vi "Get Trigger Source.vi"(8 "error in":errorcluster, 11 "VISA resource name in":refnum<visa-resource-name>) -> (0 "error out":errorcluster, 2 "Trigger Source":string, 3 "VISA resource name out":refnum<visa-resource-name>)   [LabVIEW 2021, in "Keysight U1282A.lvlib"]
doc: "El comando obtener fuente de disparo (TRIG:SOUR?) regresa el tipo de fuente de disparo."
uses:
  Keysight U1282A.lvlib
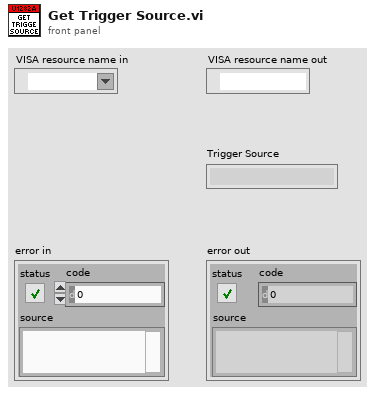
[diagram p1: front panel]
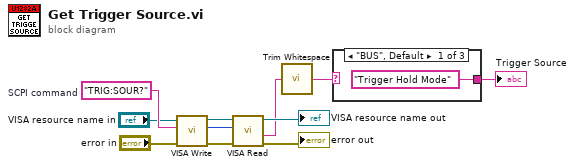
[diagram p0: block diagram]
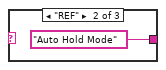
[diagram p2: hidden frame]
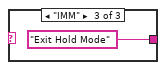
[diagram p3: hidden frame]
diagram:
  w4 = "TRIG:SOUR?"  # SCPI command
  n1 = call "VISA Write.vi"("error in"="error in", "SCPI command"=w4, "VISA resource in"="VISA resource name in") -> ("error out"=w11:errorcluster, "Bytes at Port out"=w9:u32, "VISA resource out"=w10:refnum<visa-resource-name>)  [unwired: 6 in]
  n2 = call "VISA Read.vi"("error in"=w11, "Bytes at Port in"=w9, "VISA resource in"=w10) -> ("error out"=→"error out":errorcluster, "Reading"=w3:string, "VISA resource out"=→"VISA resource name out":refnum<visa-resource-name>)  [unwired: 5 in, 1 out]
  n3 = call <vilib>:"Trim Whitespace.vi"("string"=w3) -> ("trimmed string"=w2:string)  [unwired: 1 in]
  n4 = case shown="\"BUS\", Default" w2 {
    tunnel: ["Trigger Hold Mode" "Auto Hold Mode" "Exit Hold Mode"] -> w5
    frame "BUS", Default {
    }
    frame "REF" {
    }
    frame "IMM" {
    }
  }
  "Trigger Source" <- w5
